vi "wpopup.vi"() -> ()   [LabVIEW 2014]
doc: "Target VI used in conjunction with the asynchronous call examples."
uses:
  subVI/departure.vi
  subVI/Destination.vi
  <vilib>/httpClient/LabVIEWHTTPClient.lvlib
panel:
  out "연결된 문자열 2":string
  out "departure":string
  out "Destination":string
  in  "닫기":bool
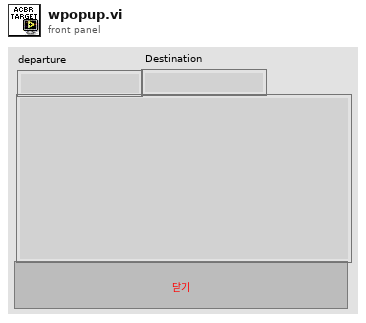
[diagram p1: front panel]
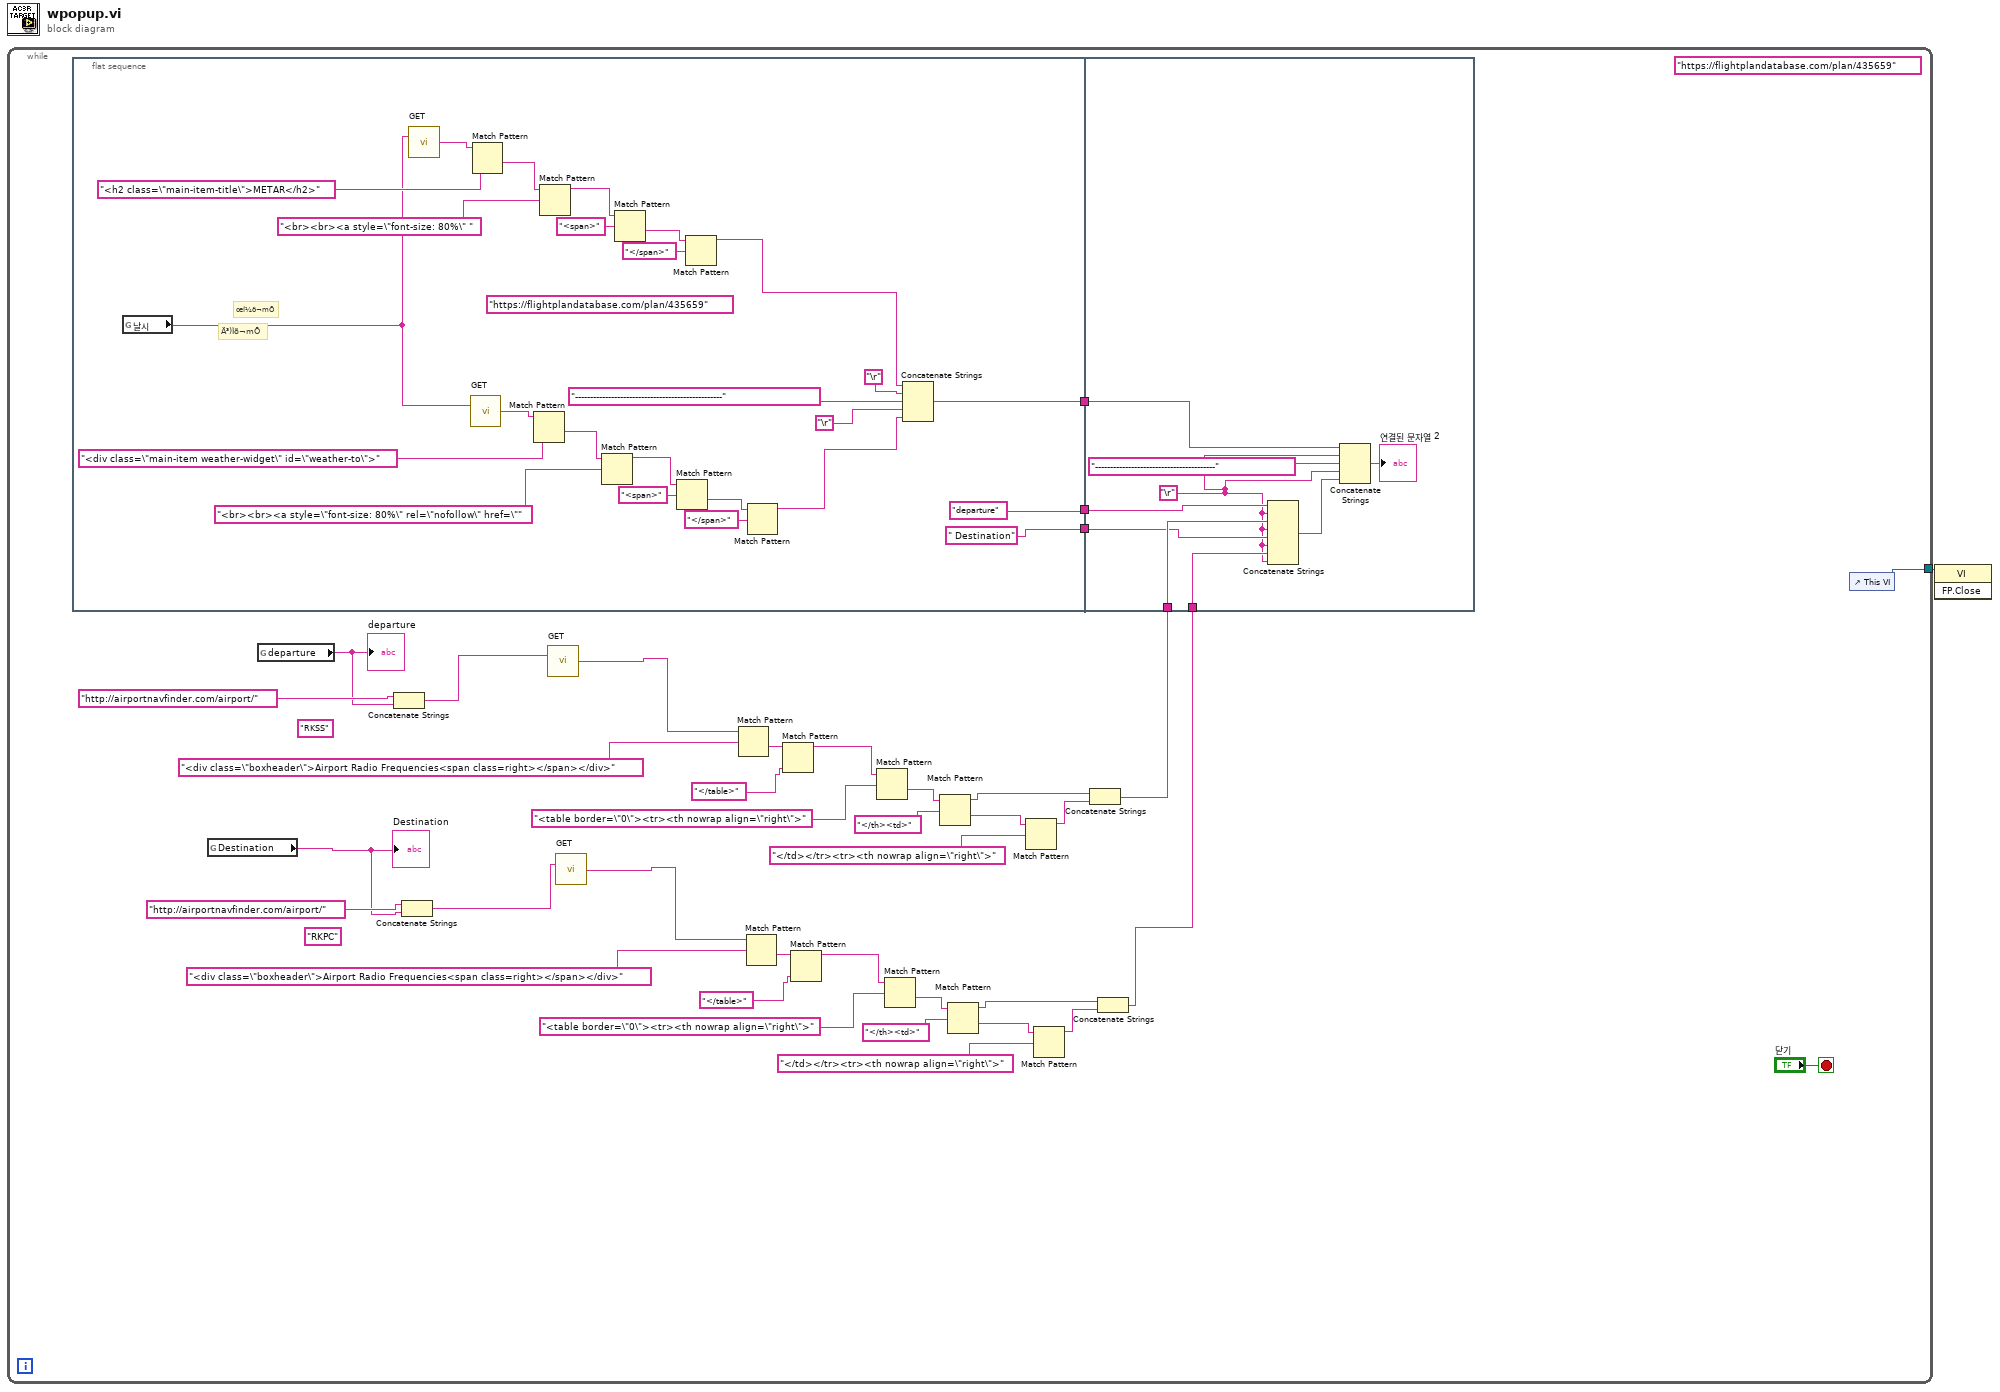
[diagram p0: block diagram]
diagram:
  n1 = while {
    tunnel: [w37] -> w1
    stop <- "닫기" stop-if-true
    (unwired) "RKPC" ("문자열")
    (unwired) "RKSS" ("문자열")
    (unwired) "https://flightplandatabase.com/plan/435659"
    n2 = flat-sequence {
      tunnel: [w41] -> w36
      tunnel: ["departure"] -> w5
      tunnel: [" Destination"] -> w4
      tunnel: w36 -> [w72]
      tunnel: w7 -> [w67]
      tunnel: w6 -> [w65]
      tunnel: w5 -> [w68]
      tunnel: w4 -> [w66]
      frame #0 {
        (unwired) "https://flightplandatabase.com/plan/435659"
        # "œÍ¼õ¬mÕ"
        # "Ä³)Ìõ¬mÕ"
        n3 = global read "날시.vi" "날시"() -> (w47:string)
        n4 = call <vilib>:"GET.vi"("url"=w47) -> ("body"=w63:string)  [unwired: 11 in, 3 out]
        n5 = call <vilib>:"GET.vi"("url"=w47) -> ("body"=w48:string)  [unwired: 11 in, 3 out]
        n6 = Match Pattern(string=w63, regular expression="<h2 class=\"main-item-title\">METAR</h2>" ("정규식")) -> (after substring=w61:string)  [unwired: 1 in, 3 out]
        n7 = Match Pattern(string=w48, regular expression="<div class=\"main-item weather-widget\" id=\"weather-to\">" ("정규식")) -> (after substring=w50:string)  [unwired: 1 in, 3 out]
        n8 = Match Pattern(string=w61, regular expression="<br><br><a style=\"font-size: 80%\" " ("정규식")) -> (before substring=w59:string)  [unwired: 1 in, 3 out]
        n9 = Match Pattern(string=w50, regular expression="<br><br><a style=\"font-size: 80%\" rel=\"nofollow\" href=\"" ("정규식")) -> (before substring=w52:string)  [unwired: 1 in, 3 out]
        n10 = Match Pattern(string=w59, regular expression="<span>" ("정규식")) -> (after substring=w57:string)  [unwired: 1 in, 3 out]
        n11 = Match Pattern(string=w52, regular expression="<span>" ("정규식")) -> (after substring=w54:string)  [unwired: 1 in, 3 out]
        n12 = Match Pattern(string=w57, regular expression="</span>" ("정규식")) -> (before substring=w43:string)  [unwired: 1 in, 3 out]
        n13 = Match Pattern(string=w54, regular expression="</span>" ("정규식")) -> (before substring=w44:string)  [unwired: 1 in, 3 out]
        n14 = Concatenate Strings(w43, "\r", "-------------------------------------------------" ("문자열"), "\r", w44) -> (w41:string)
      }
      frame #1 {
        w64 = "\r"
        n15 = Concatenate Strings(w68, w64, w67, w64, w66, w64, w65, w64) -> (w70:string)
        n16 = Concatenate Strings(w72, w64, "----------------------------------------" ("문자열"), w64, w70) -> (→"연결된 문자열 2":string)
      }
    }
    n17 = global read "Destination.vi" "Destination"() -> (w2:string)
    "Destination" <- w2
    n18 = global read "departure.vi" "departure"() -> (w3:string)
    "departure" <- w3
    n19 = Concatenate Strings("http://airportnavfinder.com/airport/", w3) -> (w35:string)
    n20 = Concatenate Strings("http://airportnavfinder.com/airport/", w2) -> (w9:string)
    n21 = call <vilib>:"GET.vi"("url"=w35) -> ("body"=w33:string)  [unwired: 11 in, 3 out]
    n22 = call <vilib>:"GET.vi"("url"=w9) -> ("body"=w11:string)  [unwired: 11 in, 3 out]
    n23 = Match Pattern(string=w33, regular expression="<div class=\"boxheader\">Airport Radio Frequencies<span class=right></span></div>" ("정규식")) -> (after substring=w31:string)  [unwired: 1 in, 3 out]
    n24 = Match Pattern(string=w11, regular expression="<div class=\"boxheader\">Airport Radio Frequencies<span class=right></span></div>" ("정규식")) -> (after substring=w13:string)  [unwired: 1 in, 3 out]
    n25 = Match Pattern(string=w31, regular expression="</table>" ("정규식")) -> (before substring=w29:string)  [unwired: 1 in, 3 out]
    n26 = Match Pattern(string=w13, regular expression="</table>" ("정규식")) -> (before substring=w8:string)  [unwired: 1 in, 3 out]
    n27 = Match Pattern(string=w29, regular expression="<table border=\"0\"><tr><th nowrap align=\"right\">" ("정규식")) -> (after substring=w27:string)  [unwired: 1 in, 3 out]
    n28 = Match Pattern(string=w8, regular expression="<table border=\"0\"><tr><th nowrap align=\"right\">" ("정규식")) -> (after substring=w16:string)  [unwired: 1 in, 3 out]
    n29 = Match Pattern(string=w27, regular expression="</th><td>" ("정규식")) -> (before substring=w23:string, after substring=w25:string)  [unwired: 1 in, 2 out]
    n30 = Match Pattern(string=w16, regular expression="</th><td>" ("정규식")) -> (before substring=w20:string, after substring=w18:string)  [unwired: 1 in, 2 out]
    n31 = Match Pattern(string=w25, regular expression="</td></tr><tr><th nowrap align=\"right\">" ("정규식")) -> (before substring=w22:string)  [unwired: 1 in, 3 out]
    n32 = Match Pattern(string=w18, regular expression="</td></tr><tr><th nowrap align=\"right\">" ("정규식")) -> (before substring=w21:string)  [unwired: 1 in, 3 out]
    n33 = Concatenate Strings(w23, w22) -> (w7:string)
    n34 = Concatenate Strings(w20, w21) -> (w6:string)
    n35 = control-ref of="This VI"() -> (w37:refnum<vi>)
  }
  n36 = invoke class="VI" method="FP.Close"(reference=w1) -> ()  [unwired: 2 in, 3 out]
